vi "CameraInputsRegulator.vi"(0 "Distance[m]":dbl, 1 "Angle(servo)":dbl) -> (2 "Fixed Height[m]":dbl, 3 "Fixed Distance[m]":dbl, 4 "Fixed Angle[deg]":dbl)   [LabVIEW 2011]
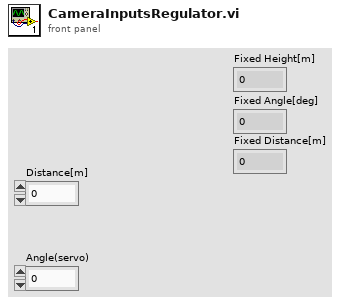
[diagram p1: front panel]
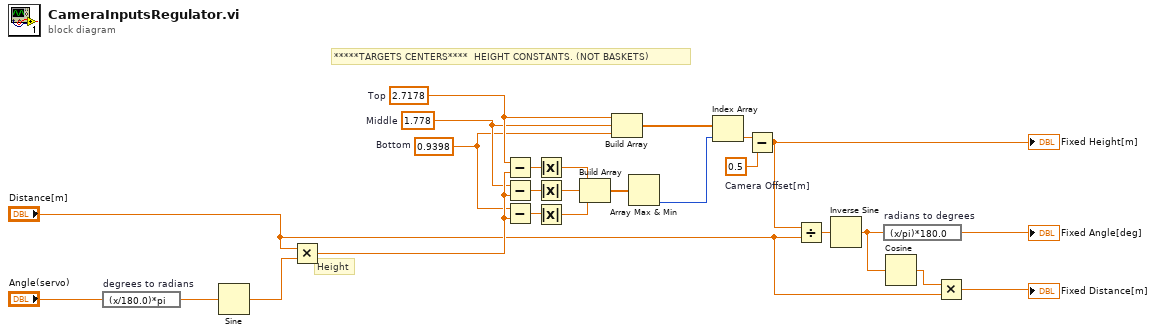
[diagram p0: block diagram]
diagram:
  w1 = 0.5  # Camera Offset[m]
  w16 = 0.9398  # Bottom
  w17 = 1.778  # Middle
  w18 = 2.7178  # Top
  # "*****TARGETS CENTERS****  HEIGHT CONSTANTS. (NOT BASKETS)"
  # "Height"
  n1 = expression code="(x/180.0)*pi" "degrees to radians"("Angle(servo)") -> (w24:dbl)
  n2 = Sine(x=w24) -> (sin(x)=w23:dbl)
  n3 = Multiply(x="Distance[m]", y=w23) -> (x*y=w22:dbl)
  n4 = Subtract(x=w18, y=w22) -> (x-y=w21:dbl)
  n5 = Subtract(x=w17, y=w22) -> (x-y=w20:dbl)
  n6 = Subtract(x=w16, y=w22) -> (x-y=w19:dbl)
  n7 = Absolute Value(x=w21) -> (abs(x)=w15:dbl)
  n8 = Absolute Value(x=w20) -> (abs(x)=w14:dbl)
  n9 = Absolute Value(x=w19) -> (abs(x)=w13:dbl)
  n10 = Build Array(w15, w14, w13) -> (w12:dbl[])
  n11 = Build Array(w18, w17, w16) -> (w11:dbl[])
  n12 = Array Max & Min(array=w12) -> (min index (indices)=w10:i32)  [unwired: 3 out]
  n13 = Index Array(array=w11, index=w10) -> (element=w3:dbl)
  n14 = Subtract(x=w3, y=w1) -> (x-y=w2:dbl)
  "Fixed Height[m]" <- w2
  n15 = Divide(x=w2, y="Distance[m]") -> (x/y=w9:dbl)
  n16 = Inverse Sine(1:w9) -> (0:w7:dbl)
  n17 = expression code="(x/pi)*180.0" "radians to degrees"(w7) -> (→"Fixed Angle[deg]":dbl)
  n18 = Cosine(x=w7) -> (cos(x)=w6:dbl)
  n19 = Multiply(x=w6, y="Distance[m]") -> (x*y=→"Fixed Distance[m]":dbl)
